vi "To String Array.vi"(8 "error in (no error)":errorcluster, 11 "Wait Step Config in":refnum<class "Wait Step Config.lvclass">) -> (0 "error out":errorcluster, 1 "Step String Array":string[](array[string]), 3 "Wait Step Config out":refnum<class "Wait Step Config.lvclass">)   [LabVIEW 2015, in "Wait Step Config.lvclass"]
uses:
  Wait Step Config.lvclass
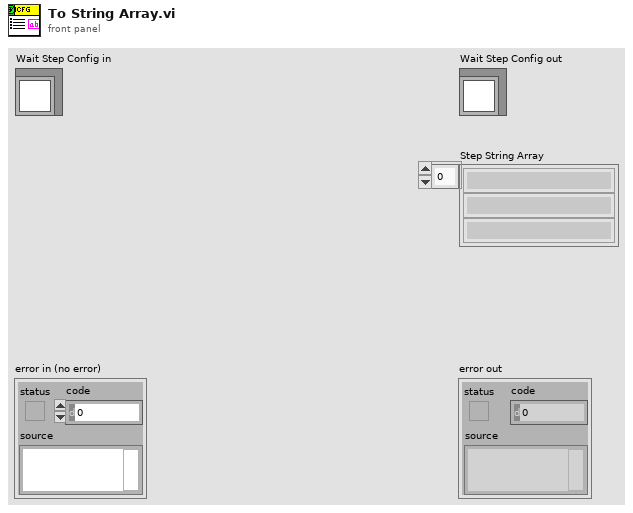
[diagram p1: front panel]
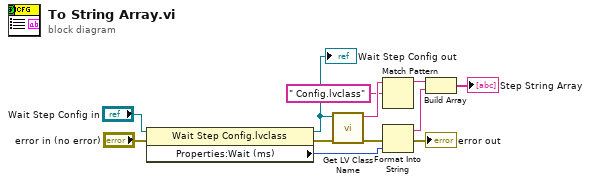
[diagram p0: block diagram]
diagram:
  n1 = property class="Wait Step Config.lvclass"(reference="Wait Step Config in", error in="error in (no error)") -> (reference out=w9:refnum<class "Wait Step Config.lvclass">, error out=w6:errorcluster, "Properties:Wait (ms)"=w11:u32)
  "Wait Step Config out" <- w9
  n2 = call <vilib>:"Get LV Class Name.vi"("error in (no error)"=w6, "object"=w9) -> ("error out"=w5:errorcluster, "class name"=w3:string)  [unwired: 8 in]
  n3 = Match Pattern(string=w3, regular expression=" Config.lvclass") -> (before substring=w2:string)  [unwired: 1 in, 3 out]
  n4 = Format Into String(error in=w5, w11) -> (resulting string=w10:string, error out=→"error out":errorcluster)  [unwired: 2 in]
  n5 = Build Array(w2, w10) -> (→"Step String Array":string[])
